vi "gun_input_diagnostics.vi"(10 "Voltage":dbl, 11 "IDG Const":T1) -> (3 "IDG State":T2)   [LabVIEW 2011]
uses:
  idg_trust_t.ctl
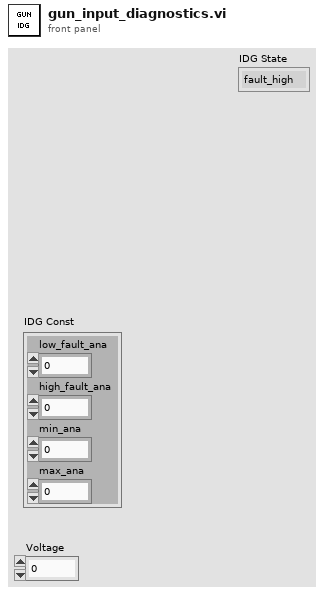
[diagram p1: front panel]
types:
  T1 = cluster{"low_fault_ana":dbl, "high_fault_ana":dbl, "min_ana":dbl, "max_ana":dbl}
  T2 = typedef "idg_trust_t.ctl" = enum16{"fault_high", "fault_low", "out_high", "out_low", "trust"}
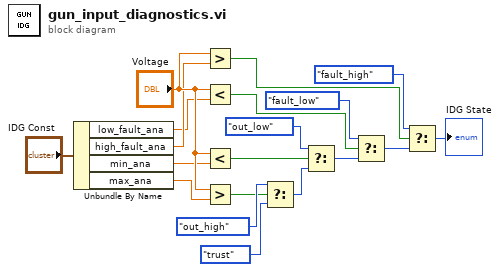
[diagram p0: block diagram]
diagram:
  n1 = Unbundle By Name("IDG Const") -> ("low_fault_ana"=w3:dbl, "high_fault_ana"=w5:dbl, "min_ana"=w9:dbl, "max_ana"=w14:dbl)
  n2 = Greater?(x="Voltage", y=w5) -> (0:w6:bool)
  n3 = Less?(x="Voltage", y=w3) -> (x < y?=w2:bool)
  n4 = Less?(x="Voltage", y=w9) -> (x < y?=w12:bool)
  n5 = Greater?(x="Voltage", y=w14) -> (0:w15:bool)
  n6 = Select(t=idg_trust_t."out_high", s=w15, f=idg_trust_t."trust" ("t")) -> (s? t:f=w16:T2)
  n7 = Select(t=idg_trust_t."out_low", s=w12, f=w16) -> (s? t:f=w10:T2)
  n8 = Select(t=idg_trust_t."fault_low", s=w2, f=w10) -> (s? t:f=w7:T2)
  n9 = Select(t=idg_trust_t."fault_high", s=w6, f=w7) -> (s? t:f=→"IDG State":T2)
